vi "Get Socket Count.vi"(8 "error in (no error)":errorcluster, 11 "Teststand in":refnum<class "Teststand.lvclass">) -> (0 "error out":errorcluster, 2 "Socket Count":i16, 3 "Teststand out":refnum<class "Teststand.lvclass">)   [LabVIEW 2023, in "HardwareAbstractionLayer_LVOOP.lvlib" / "Teststand.lvclass"]
doc: "This vi used get teststand total socket count"
uses:
  Teststand.lvclass
  Teststand.lvclass/Teststand.ctl
  <vilib>/addons/TestStand/_TSUtility.llb/TestStand - Get Property Value (Number {Signed 16-bit Integer}).vi
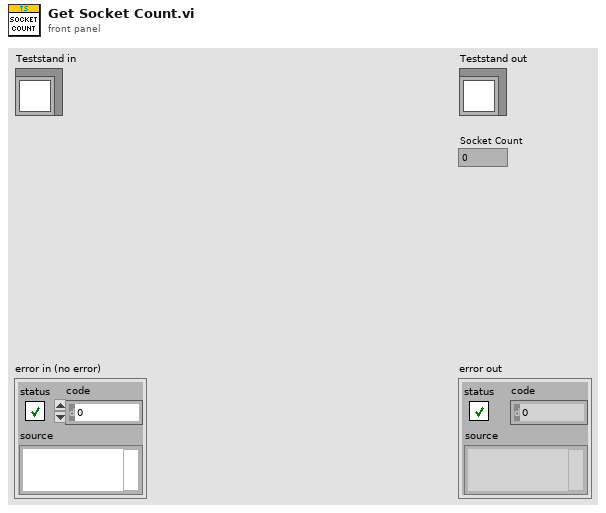
[diagram p1: front panel]
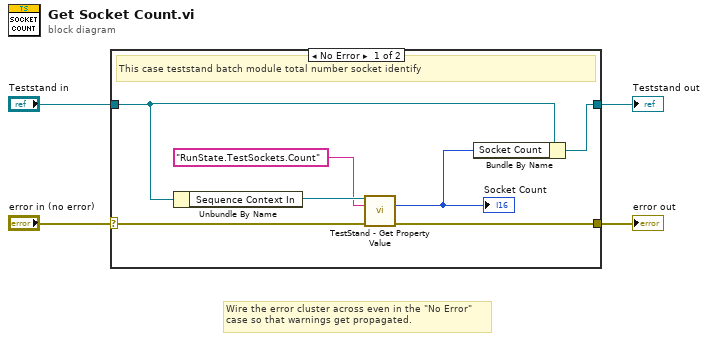
[diagram p0: block diagram]
diagram:
  # "Wire the error cluster across even in the \"No Error\"\ncase so that warnings get propagated."
  n1 = case shown="No Error" "error in (no error)" {
    selector: "error in (no error)" -> [w10 w13]
    tunnel: [w9 w13] -> w3
    tunnel: [w6 w12] -> w1
    tunnel: "Teststand in" -> [w7 w12]
    frame No Error {
      # "This case teststand batch module total number socket identify"
      n2 = Unbundle By Name(w7) -> ("Sequence Context In"=w11:refnum<k7>)
      n3 = call-poly <vilib>:"TestStand - Get Property Value.vi"("Sequence Context In"=w11, "Lookup String"="RunState.TestSockets.Count", "error in (no error)"=w10) -> ("Value"=w5:i16, "error out"=w9:errorcluster)  [unwired: 10 in, 1 out]
      "Socket Count" <- w5
      n4 = Bundle By Name(cluster=w7, "Socket Count"=w5) -> (w6:refnum<class "Teststand.lvclass">)
    }
    frame Error {
    }
  }
  "error out" <- w3
  "Teststand out" <- w1
